vi "Close.vi"(8 "error in":errorcluster, 11 "HSU MCU V2 Monitor CFG in":refnum<class "HSU MCU V2 Monitor CFG.lvclass">) -> (0 "error out":errorcluster, 3 "HSU MCU V2 Monitor CFG out":refnum<class "HSU MCU V2 Monitor CFG.lvclass">)   [LabVIEW 2023, in "HSU MCU V2 Monitor CFG.lvclass"]
uses:
  HSU MCU V2 Monitor CFG.lvclass
  HSU MCU V2 Monitor CFG.lvclass/HSU MCU V2 Monitor CFG.ctl
  Interfaces/IConfigure/IConfigure.lvclass
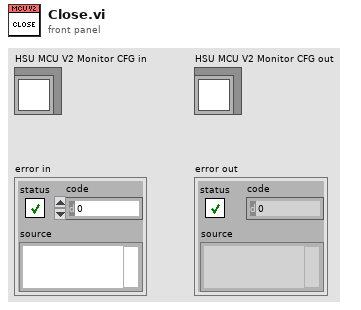
[diagram p1: front panel]
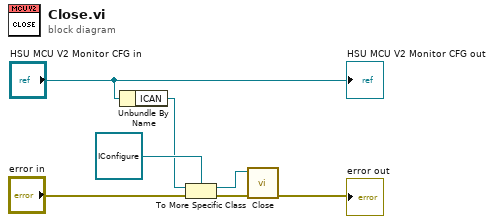
[diagram p0: block diagram]
diagram:
  n1 = Unbundle By Name("HSU MCU V2 Monitor CFG in") -> ("ICAN"=w4:refnum<class "ICAN.lvclass">)
  n2 = To More Specific Class(target class=refnum<class "IConfigure.lvclass"> refnum ("IConfigure.lvclass"), reference=w4, error in="error in") -> (specific class reference=w1:refnum<class "IConfigure.lvclass">, error out=w3:errorcluster)
  n3 = call-dynamic "Close.vi"("error in"=w3, "IConfigure in"=w1) -> ("error out"=→"error out":errorcluster)  [unwired: 8 in, 1 out]
  "HSU MCU V2 Monitor CFG out" <- "HSU MCU V2 Monitor CFG in"
